vi "Response.vi"(8 "error in":errorcluster, 11 "System Data":T1={"System"={"Active"=FALSE, "Exit"=FALSE, "Command wait"="", "Status_Time"=0, "Time_GPS"=0}, "Stepper Motor"={"Connection Reference"="", "Valid Connection"=FALSE, "Speed"=15}, "Camera Data"={"Image path"=path "", "Filenames"=[], "Filenames queue"=[]}, "Core"={"Close Panel on Exit?"=FALSE, "Current VI Reference"=refnum}} {"Stepper Motor"."Speed" scale=0.0..30.0}) -> (0 "error out":errorcluster, 1 "GPS Status":bool, 2 "next state":string, 3 "System Data out":T1={"System"={"Active"=FALSE, "Exit"=FALSE, "Command wait"="", "Status_Time"=0, "Time_GPS"=0}, "Stepper Motor"={"Connection Reference"="", "Valid Connection"=FALSE, "Speed"=15}, "Camera Data"={"Image path"=path "", "Filenames"=[], "Filenames queue"=[]}, "Core"={"Close Panel on Exit?"=FALSE, "Current VI Reference"=refnum}} {"Stepper Motor"."Speed" scale=0.0..30.0}, 4 "Data":string[][](array[string]), 6 "NewData":bool)   [LabVIEW 2019]
uses:
  System Data.ctl
  Stepper Data.ctl
  Camera Data.ctl
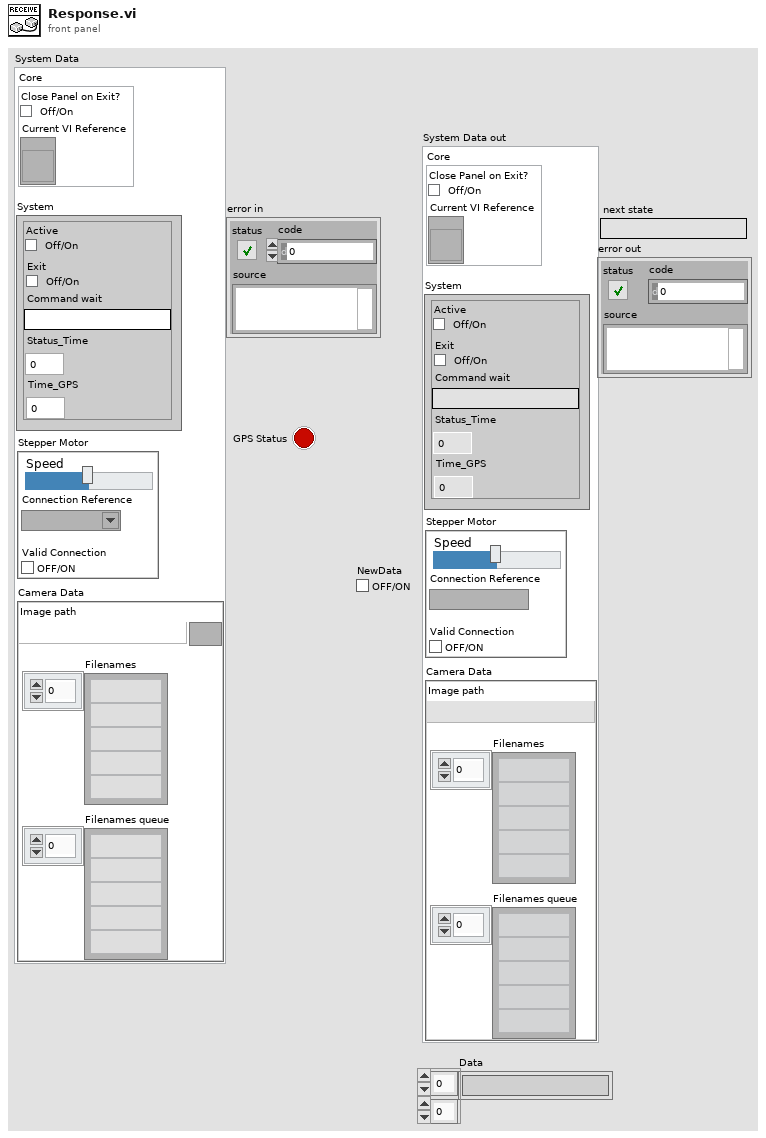
[diagram p1: front panel]
types:
  T1 = typedef "System Data.ctl" = cluster{"System":cluster{"Active":bool, "Exit":bool, "Command wait":string, "Status_Time":i32, "Time_GPS":i32}, "Stepper Motor":T2, "Camera Data":T3, "Core":cluster{"Close Panel on Exit?":bool, "Current VI Reference":refnum<vi>}}
  T2 = typedef "Stepper Data.ctl" = cluster{"Connection Reference":refnum<visa-resource-name>, "Valid Connection":bool, "Speed":i32}
  T3 = typedef "Camera Data.ctl" = cluster{"Image path":path, "Filenames":string[], "Filenames queue":string[]}
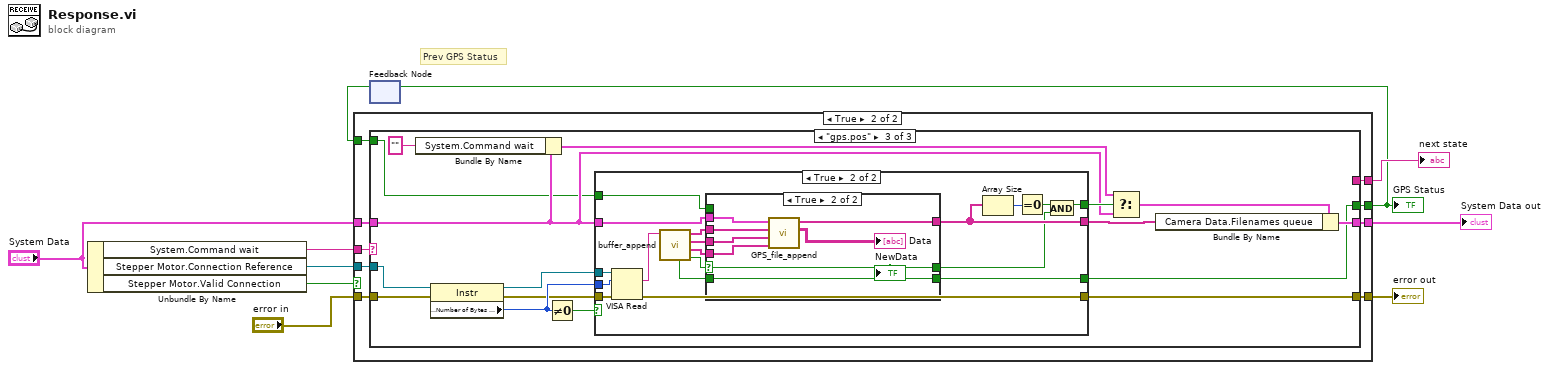
[diagram p0: block diagram]
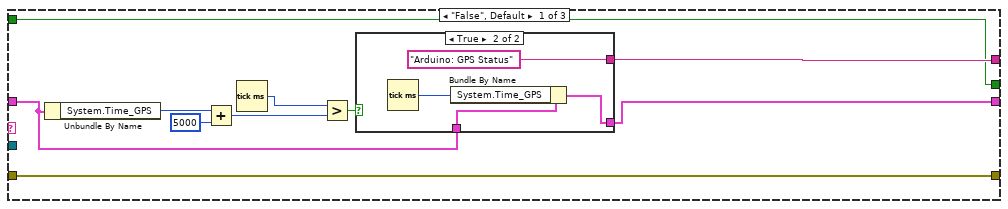
[diagram p3: hidden frame]
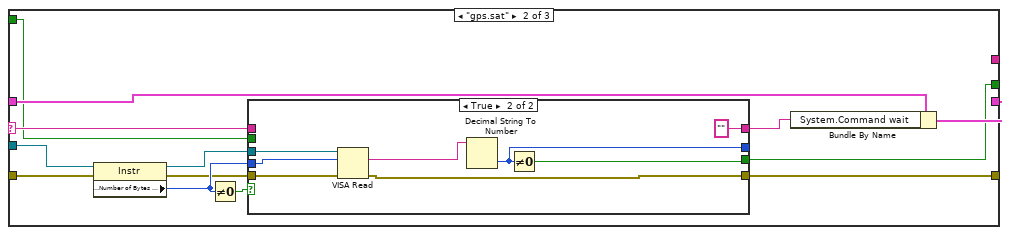
[diagram p5: hidden frame]
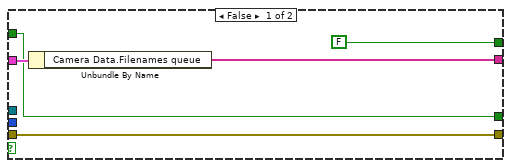
[diagram p7: hidden frame]
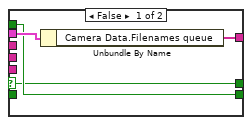
[diagram p8: hidden frame]
diagram:
  # "Prev GPS Status"
  n1 = Unbundle By Name("System Data") -> ("System.Command wait"=w5:string, "Stepper Motor.Connection Reference"=w4:refnum<visa-resource-name>, "Stepper Motor.Valid Connection"=w1:bool)
  n2 = feedback #1() -> (w2:bool)  [unwired: 1 in]
  n3 = case shown="True" w1 {
    tunnel: [w14 w23] -> w10
    tunnel: [w13 w22] -> w9
    tunnel: "error in" -> [w11 w21]
    tunnel: [w11 w20] -> w7
    tunnel: "System Data" -> [w14 w19]
    tunnel: w5 -> [w13 w18]
    tunnel: w4 -> [_ w17]
    tunnel: [w12 w16] -> w3
    tunnel: w2 -> [w12 w15]
    frame False {
    }
    frame True {
      n4 = case shown="\"gps.pos\"" w18 {
        selector: w18 -> [_ w40 _]
        tunnel: w17 -> [_ w47 w74]
        tunnel: w21 -> [w32 w46 w73]
        tunnel: [w32 w45 w72] -> w20
        tunnel: w19 -> [w25 w44 w66]
        tunnel: [w24 w43 w67] -> w23
        tunnel: [w33 _ _] -> w22
        tunnel: [w27 w42 w64] -> w16
        tunnel: w15 -> [w27 w39 w63]
        frame "False", Default {
          n5 = Unbundle By Name(w25) -> ("System.Time_GPS"=w26:i32)
          n6 = Add(x=w26, y=u32 5000) -> (x+y=w28:u32)
          n7 = Tick Count (ms)() -> (millisecond timer value=w31:u32)
          n8 = Greater?(x=w31, y=w28) -> (0:w30:bool)
          n9 = case shown="True" w30 {
            tunnel: [_ "Arduino: GPS Status"] -> w33
            tunnel: w25 -> [w34 w37]
            tunnel: [w34 w35] -> w24
            frame False {
            }
            frame True {
              n10 = Tick Count (ms)() -> (millisecond timer value=w36:u32)
              n11 = Bundle By Name(cluster=w37, "System.Time_GPS"=w36) -> (w35:T1)
            }
          }
        }
        frame "gps.sat" {
          n12 = property class="Instr"(reference=w47, error in=w46) -> (reference out=w49:refnum<visa-resource-name>, error out=w50:errorcluster, "Serial Settings:Number of Bytes at Serial Port"=w51:u32)
          n13 = Not Equal To 0?(x=w51) -> (x != 0?=w48:bool)
          n14 = case shown="True" w48 {
            tunnel: w49 -> [_ w62]
            tunnel: w51 -> [_ w61]
            tunnel: [w52 w59] -> w42
            tunnel: w50 -> [w54 w58]
            tunnel: [w54 w57] -> w45
            tunnel: [_ w56] -> _
            tunnel: [w53 "" ("System.Command wait")] -> w41
            tunnel: w40 -> [w53 _]
            tunnel: w39 -> [w52 _]
            frame False {
            }
            frame True {
              n15 = VISA Read(VISA resource name=w62, byte count=w61, error in (no error)=w58) -> (read buffer=w60:string, error out=w57:errorcluster)  [unwired: 2 out]
              n16 = Decimal String To Number(string=w60) -> (number=w56:i32)  [unwired: 2 in, 1 out]
              n17 = Not Equal To 0?(x=w56) -> (x != 0?=w59:bool)
            }
          }
          n18 = Bundle By Name(cluster=w44, "System.Command wait"=w41) -> (w43:T1)
        }
        frame "gps.pos" {
          n19 = Bundle By Name(cluster=w66, "System.Command wait"="") -> (w70:T1)
          n20 = property class="Instr"(reference=w74, error in=w73) -> (reference out=w76:refnum<visa-resource-name>, error out=w77:errorcluster, "Serial Settings:Number of Bytes at Serial Port"=w78:u32)
          n21 = Not Equal To 0?(x=w78) -> (x != 0?=w75:bool)
          n22 = case shown="True" w75 {
            tunnel: w76 -> [_ w101]
            tunnel: w78 -> [_ w100]
            tunnel: w77 -> [w83 w99]
            tunnel: [w83 w98] -> w72
            tunnel: [FALSE w85] -> w69
            tunnel: w66 -> [w81 w97]
            tunnel: [w80 w93] -> w65
            tunnel: [w79 w88] -> w64
            tunnel: w63 -> [w79 w86]
            frame False {
              n23 = Unbundle By Name(w81) -> ("Camera Data.Filenames queue"=w80:string[])
            }
            frame True {
              n24 = VISA Read(VISA resource name=w101, byte count=w100, error in (no error)=w99) -> (read buffer=w94:string, error out=w98:errorcluster)  [unwired: 2 out]
              n25 = call "buffer_append.vi"("read buffer"=w94) -> ("Received?"=w90:bool, "Alt"=w89:string[], "Lng"=w95:string[], "Lat"=w96:string[], "GPS Valid?"=w87:bool)  [unwired: 6 in]
              n26 = case shown="True" w90 {
                selector: w90 -> [w102 w107]
                tunnel: w97 -> [w105 w113]
                tunnel: w96 -> [_ w111]
                tunnel: w95 -> [_ w110]
                tunnel: [w104 w112] -> w93
                tunnel: w89 -> [_ w109]
                tunnel: [w103 w108] -> w88
                tunnel: w87 -> [_ w108]
                tunnel: w86 -> [w103 _]
                tunnel: [w102 w107] -> w84
                frame False {
                  n27 = Unbundle By Name(w105) -> ("Camera Data.Filenames queue"=w104:string[])
                }
                frame True {
                  n28 = call "GPS_file_append.vi"("Alt"=w109, "Lng"=w110, "Lat"=w111, "input cluster"=w113) -> ("Data"=→"Data":string[][], "Filenames queue"=w112:string[])  [unwired: 6 in]
                  "NewData" <- w107
                }
              }
              n29 = Array Size(array=w93) -> (size(s)=w92:i32)
              n30 = Equal To 0?(x=w92) -> (x = 0?=w91:bool)
              n31 = And(x=w91, y=w84) -> (x .and. y?=w85:bool)
            }
          }
          n32 = Select(t=w70, s=w69, f=w66) -> (s? t:f=w68:T1)
          n33 = Bundle By Name(cluster=w68, "Camera Data.Filenames queue"=w65) -> (w67:T1)
        }
      }
    }
  }
  "System Data out" <- w10
  "next state" <- w9
  "error out" <- w7
  "GPS Status" <- w3
  n34 = feedback-in #1(w3) -> ()
